vi "save_read_script.vi"(2 "w-r":enum16{"save", "read"}(ring), 3 "intput table":string[][](array[string])=[["dede", ""], ["", "ddddd"]]) -> (0 "error out":errorcluster, 1 "output table":string[][](array[string]))   [LabVIEW 2026]
uses:
  <vilib>/Utility/NIReport.llb/Report Type.ctl
  <vilib>/Utility/file.llb/Write Delimited Spreadsheet (string).vi
  <vilib>/Utility/NIReport.llb/Append Text Table to Report (wrap).vi
  <vilib>/addons/_office/excel.llb/Excel Get Data ([str]).vi
  <vilib>/Utility/NIReport.llb/NI_report.lvclass
  <vilib>/Utility/NIReport.llb/NI_ReportGenerationCore.lvlib
  <vilib>/Utility/NIReport.llb/Excel/NI_Excel.lvclass
  <vilib>/addons/_office/NI_ReportGenerationToolkit.lvlib
  <vilib>/Utility/file.llb/Read Delimited Spreadsheet (string).vi
panel:
  in  "csv-excel":enum16{"csv", "excel"}(ring)
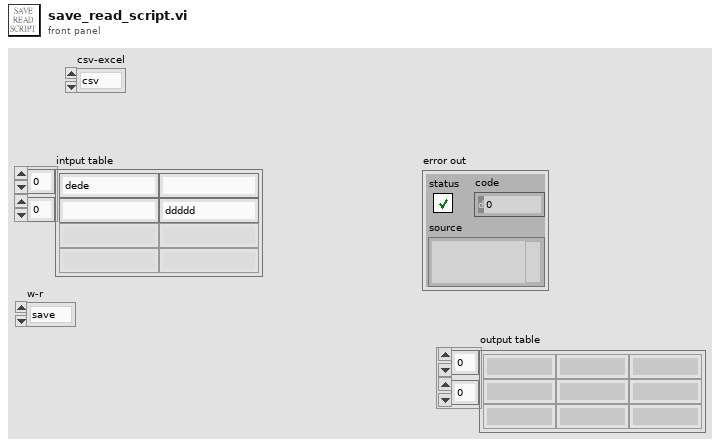
[diagram p1: front panel]
types:
  T1 = typedef "NI_ReportGenerationCore.lvlib/Report Type.ctl" = enum16{"HTML", "Word", "Excel"}
  T2 = enum16{"maximized", "minimized", "normal", "no change"}
  T3 = enum16{"Standard Report", "HTML", "Word", "Excel"}
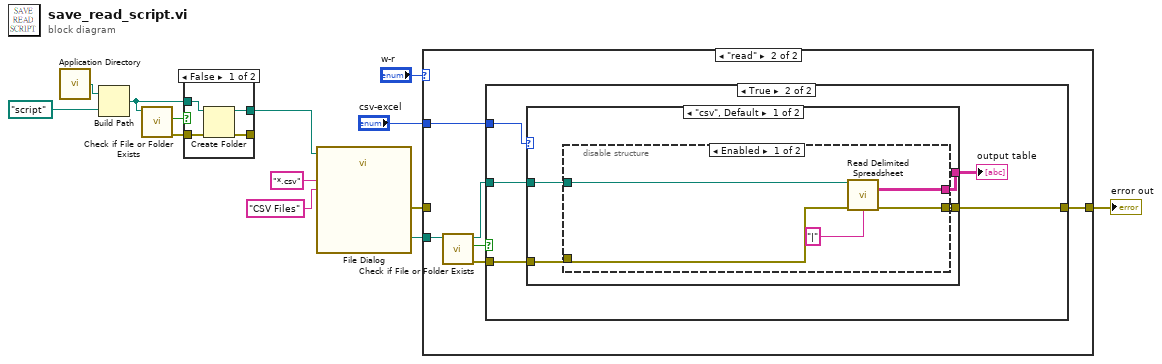
[diagram p0: block diagram]
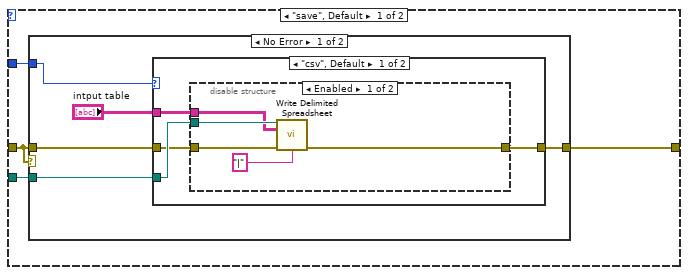
[diagram p3: hidden frame]
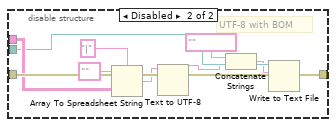
[diagram p4: hidden frame]
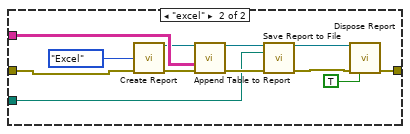
[diagram p5: hidden frame]
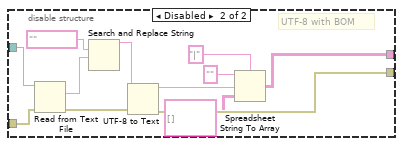
[diagram p8: hidden frame]
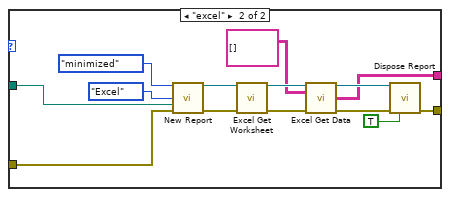
[diagram p9: hidden frame]
diagram:
  n1 = call <vilib>:"Application Directory.vi"() -> ("Application Directory"=w13:path)
  n2 = Build Path(base path=w13, name or relative path=path "script") -> (appended path=w7:path)
  n3 = call <vilib>:"Check if File or Folder Exists.vi"("path"=w7) -> ("error out"=w9:errorcluster, "file or folder exists?"=w8:bool)  [unwired: 8 in, 1 out]
  n4 = case shown="False" w8 {
    tunnel: w7 -> [w17 w19]
    tunnel: [w16 w19] -> w1
    tunnel: w9 -> [w15 w18]
    tunnel: [w14 w18] -> _
    frame False {
      n5 = Create Folder(path (use dialog)=w17, error in=w15) -> (created path=w16:path, error out=w14:errorcluster)  [unwired: 1 in, 1 out]
    }
    frame True {
    }
  }
  n6 = call "File Dialog"("start path"=w1, "pattern (all files)"="*.csv", "pattern label"="CSV Files" ("pattern (all files)")) -> ("selected path"=w3:path, "error out"=w2:errorcluster)  [unwired: 9 in, 2 out]
  n7 = case shown="\"read\"" "w-r" {
    tunnel: [w23 w62] -> w6
    tunnel: "csv-excel" -> [w22 w61]
    tunnel: w3 -> [w21 w60]
    tunnel: w2 -> [w20 _]
    frame "save", Default {
      n8 = case shown="No Error" w20 {
        tunnel: [w28 w59] -> w23
        tunnel: w22 -> [w27 _]
        tunnel: w20 -> [w26 w59]
        tunnel: w21 -> [w24 _]
        frame No Error {
          n9 = case shown="\"csv\", Default" w27 {
            tunnel: "intput table" -> [w31 w58]
            tunnel: w24 -> [w32 w51]
            tunnel: [w29 w48] -> w28
            tunnel: w26 -> [w30 w47]
            frame "csv", Default {
              n10 = disable-structure shown="Enabled" {
                disable-tunnel: w32 -> [w37 w41]
                disable-tunnel: w31 -> [w36 w42]
                disable-tunnel: w30 -> [w35 w46]
                disable-tunnel: [w34 w46] -> w29
                frame Enabled {
                  n11 = call-poly <vilib>:"Write Delimited Spreadsheet.vi"("file path (dialog if empty)"=w37, "2D data"=w36, "error in (no error)"=w35, "delimiter (\\t)"="|" ("delimiter (\\t)")) -> ("error out"=w34:errorcluster)  [unwired: 10 in, 1 out]
                }
                frame Disabled {
                  # "UTF-8 with BOM"
                  n12 = Array To Spreadsheet String(delimiter (Tab)="|", array=w42, 3:"" ("format string")) -> (spreadsheet string=w45:string)
                  n13 = Text to UTF-8(11:w45) -> (3:w39:string)  [unwired: 2 in, 1 out]
                  n14 = Concatenate Strings("﻿" ("format string"), w39) -> (w38:string)
                  n15 = Write to Text File(file (use dialog)=w41, text=w38) -> ()  [unwired: 2 in, 3 out]
                }
              }
            }
            frame "excel" {
              n16 = call <vilib>:"Create Report.vi"("report type"=Report_Type."Excel" ("Report Type"), "error in (no error)"=w47) -> ("report out"=w53:refnum<class "NI_report.lvclass">, "error out"=w52:errorcluster)  [unwired: 12 in]
              n17 = call-poly <vilib>:"Append Table to Report.vi"("report in"=w53, "text data"=w58, "error in (no error)"=w52) -> ("report out"=w54:refnum<class "NI_report.lvclass">, "error out"=w55:errorcluster)  [unwired: 9 in, 2 out]
              n18 = call-dynamic "Save Report to File.vi"("report in"=w54, "report file path"=w51, "error in (no error)"=w55) -> ("report out"=w57:refnum<class "NI_report.lvclass">, "error out"=w56:errorcluster)  [unwired: 11 in]
              n19 = call-dynamic "Dispose Report.vi"("report in"=w57, "error in (no error)"=w56, "close report? (T)"=TRUE ("Close Report? (T)")) -> ("error out"=w48:errorcluster)  [unwired: 12 in]
            }
          }
        }
        frame Error {
        }
      }
    }
    frame "read" {
      n20 = call <vilib>:"Check if File or Folder Exists.vi"("path"=w60) -> ("error out"=w65:errorcluster, "file or folder exists?"=w63:bool, "dup path"=w64:path)  [unwired: 8 in]
      n21 = case shown="True" w63 {
        tunnel: [w66 w71] -> w62
        tunnel: w64 -> [_ w70]
        tunnel: w65 -> [w66 w69]
        tunnel: w61 -> [_ w68]
        frame False {
        }
        frame True {
          n22 = case shown="\"csv\", Default" w68 {
            tunnel: [w74 w102] -> w71
            tunnel: w70 -> [w72 w98]
            tunnel: w69 -> [w73 w96]
            tunnel: [w75 w93] -> w67
            frame "csv", Default {
              n23 = disable-structure shown="Enabled" {
                disable-tunnel: [w79 w84] -> w75
                disable-tunnel: [w78 w87] -> w74
                disable-tunnel: w73 -> [w77 w89]
                disable-tunnel: w72 -> [w76 w86]
                frame Enabled {
                  n24 = call-poly <vilib>:"Read Delimited Spreadsheet.vi"("file path (dialog if empty)"=w76, "error in (no error)"=w77, "delimiter (\\t)"="|" ("delimiter (\\t)")) -> ("all rows"=w79:string[][], "error out"=w78:errorcluster)  [unwired: 7 in, 4 out]
                }
                frame Disabled {
                  # "UTF-8 with BOM"
                  n25 = Read from Text File(file (use dialog)=w86, error in=w89) -> (text=w82:string, error out=w88:errorcluster)  [unwired: 2 in, 2 out]
                  n26 = Search and Replace String(input string=w82, search string="﻿" ("format string")) -> (result string=w81:string)  [unwired: 6 in, 3 out]
                  n27 = UTF-8 to Text(8:w88, 11:w81) -> (0:w87:errorcluster, 3:w92:string)  [unwired: 1 in]
                  n28 = Spreadsheet String To Array(delimiter (Tab)="|", format string="", spreadsheet string=w92, array type (2D Dbl)=string[][] []) -> (array=w84:string[][])
                }
              }
            }
            frame "excel" {
              n29 = call <vilib>:"New Report.vi"("window state (normal)"=T2."minimized", "report type"=T3."Excel", "template (empty)"=w98, "error in (no error)"=w96) -> ("report out"=w105:refnum<class "NI_report.lvclass">, "error out"=w95:errorcluster)  [unwired: 10 in]
              n30 = call <vilib>:"Excel Get Worksheet.vi"("report in"=w105, "error in (no error)"=w95) -> ("report out"=w104:refnum<class "NI_report.lvclass">, "error out"=w94:errorcluster)  [unwired: 12 in]
              n31 = call-poly <vilib>:"Excel Get Data.vi"("report in"=w104, "data type"=string[][] [], "error in (no error)"=w94) -> ("report out"=w100:refnum<class "NI_report.lvclass">, "data"=w93:string[][], "error out"=w99:errorcluster)  [unwired: 10 in]
              n32 = call-dynamic "Dispose Report.vi"("report in"=w100, "error in (no error)"=w99, "close report? (T)"=TRUE ("Close Report? (T)")) -> ("error out"=w102:errorcluster)  [unwired: 12 in]
            }
          }
          "output table" <- w67
        }
      }
    }
  }
  "error out" <- w6
